vi "1C Wind Calculations.vi"(7 "Boat Heading":T3 format="%05.1f", 8 "Boat Velocity":T2 {"East" format="%#_5g"}, 9 "Absolute Wind":T2 {"East" format="%#_5g"}, 10 "Add Randomness\nTo Wind Measurement":bool) -> (1 "Apparent Wind Speed":T4, 2 "Apparent Wind\nDirection":T5, 3 "Apparent Wind":T1)   [LabVIEW 2011]
doc: "Given absolute wind, boat velocity and heading, produces apparent wind data. Also places this data on the global."
uses:
  2-Think/2 Typedefs/Velocity.ctl
  2-Think/2 Typedefs/apparent wind.ctl
  2-Think/2 Globals/2 Global.vi
  2-Think/2 Typedefs/apparent wind direction.ctl
  2-Think/2 Typedefs/apparent wind speed.ctl
  2-Think/2 Typedefs/heading.ctl
panel:
  out "Apparent Wind\nin global rotation frame":T2 {"East" format="%#_5g"}
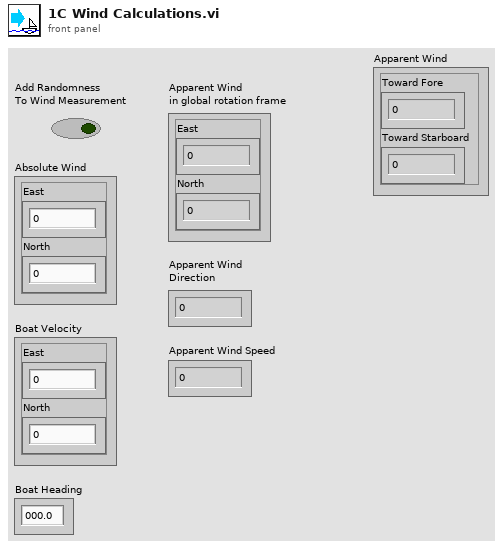
[diagram p1: front panel]
types:
  T1 = typedef "apparent wind.ctl" = cluster{"Toward Fore":dbl, "Toward Starboard":dbl}
  T2 = typedef "Velocity.ctl" = cluster{"East":dbl, "North":dbl}
  T3 = typedef "heading.ctl" = dbl
  T4 = typedef "apparent wind speed.ctl" = dbl
  T5 = typedef "apparent wind direction.ctl" = dbl
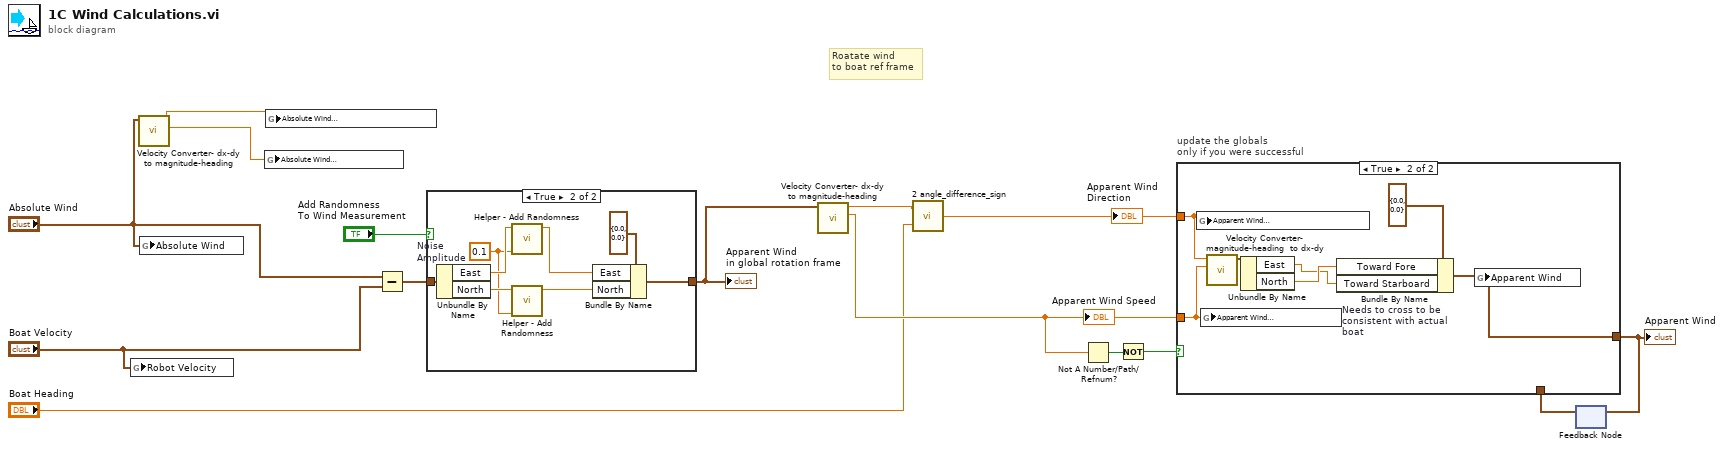
[diagram p0: block diagram]
diagram:
  # "Roatate wind\nto boat ref frame"
  n1 = global write "2 Global.vi" "Robot Velocity"("Boat Velocity") -> ()
  n2 = call "Velocity Converter- dx-dy to magnitude-heading.vi"("Vector In"="Absolute Wind") -> ("Magnitude Out"=w14:dbl, "Heading Out"=w15:T3)  [unwired: 9 in]
  n3 = global write "2 Global.vi" "Absolute Wind"("Absolute Wind") -> ()
  n4 = global write "2 Global.vi" "Absolute Wind\nSpeed"(w14) -> ()
  n5 = global write "2 Global.vi" "Absolute Wind\nDirection (º)"(w15) -> ()
  n6 = Subtract(x="Absolute Wind", y="Boat Velocity") -> (x-y=w10:T2)
  n7 = case shown="True" "Add Randomness\nTo Wind Measurement" {
    tunnel: [w16 w24] -> w7
    tunnel: w10 -> [w16 w23]
    frame False {
    }
    frame True {
      w18 = 0.1  # Noise Amplitude
      n8 = Unbundle By Name(w23) -> ("East"=w22:dbl, "North"=w21:dbl)
      n9 = call "Helper - Add Randomness.vi"("Amplitude (1)"=w18, "Numeric in"=w22) -> ("Numeric out"=w19:dbl)  [unwired: 9 in]
      n10 = call "Helper - Add Randomness.vi"("Amplitude (1)"=w18, "Numeric in"=w21) -> ("Numeric out"=w20:dbl)  [unwired: 9 in]
      n11 = Bundle By Name(cluster=T2 {"East"=0.0, "North"=0.0} ("Apparent Wind 2"), "East"=w19, "North"=w20) -> (w24:T2)
    }
  }
  "Apparent Wind\nin global rotation frame" <- w7
  n12 = call "Velocity Converter- dx-dy to magnitude-heading.vi"("Vector In"=w7) -> ("Magnitude Out"=w11:dbl, "Heading Out"=w2:T3)  [unwired: 9 in]
  "Apparent Wind Speed" <- w11
  n13 = call "2 angle_difference_sign.vi"("Angle 2"="Boat Heading", "Angle 1"=w2) -> ("Difference"=w1:dbl)
  "Apparent Wind\nDirection" <- w1
  n14 = Not A Number/Path/Refnum?(number/path/refnum=w11) -> (NaN/Path/Refnum?=w8:bool)
  n15 = Not(x=w8) -> (.not. x?=w9:bool)
  n16 = feedback #1() -> (w4:T1)  [unwired: 1 in]
  n17 = case "update the globals\nonly if you were successful" shown="True" w9 {
    tunnel: w1 -> [_ w32]
    tunnel: w11 -> [_ w31]
    tunnel: [w25 w26] -> w5
    tunnel: w4 -> [w25 _]
    frame False {
    }
    frame True {
      n18 = global write "2 Global.vi" "Apparent Wind\nDirection (º)"(w32) -> ()
      n19 = global write "2 Global.vi" "Apparent Wind\nSpeed"(w31) -> ()
      n20 = call "Velocity Converter- magnitude-heading  to dx-dy.vi"("Magnitude"=w31, "Heading"=w32) -> ("Vector Out"=w30:T2)  [unwired: 9 in]
      n21 = Unbundle By Name(w30) -> ("East"=w27:dbl, "North"=w28:dbl)
      n22 = Bundle By Name "Needs to cross to be consistent with actual boat"(cluster=T1 {"Toward Fore"=0.0, "Toward Starboard"=0.0} ("Apparent Wind"), "Toward Fore"=w28, "Toward Starboard"=w27) -> (w26:T1)
      n23 = global write "2 Global.vi" "Apparent Wind"(w26) -> ()
    }
  }
  "Apparent Wind" <- w5
  n24 = feedback-in #1(w5) -> ()
